vi "Publish Latest Data to Logger.vi"(8 "error in (no error)":errorcluster, 11 "Measurement in":refnum<class "Measurement.lvclass">) -> (0 "error out":errorcluster, 3 "Measurement out":refnum<class "Measurement.lvclass">)   [LabVIEW 2026, in "Measurement Actor.lvlib" / "Measurement.lvclass"]
uses:
  Measurement.lvclass
  Measurement.lvclass/Measurement.ctl
  Logger/Logger Messages/Write Data to File Msg/Write Data to File Msg.lvclass/Write Data to File Msg.ctl
  <vilib>/ActorFramework/Message Enqueuer/Message Enqueuer.lvclass/Message Enqueuer.ctl
  <vilib>/ActorFramework/Message Enqueuer/Enqueue.vi
  Logger/Logger Messages/Write Data to File Msg/Write Data to File Msg.lvclass
  C:/Program Files/National Instruments/LabVIEW 2026/vi.lib/ActorFramework/Message/Message.lvclass
  <vilib>/ActorFramework/Message Priority Queue/Priority Enqueue.vi
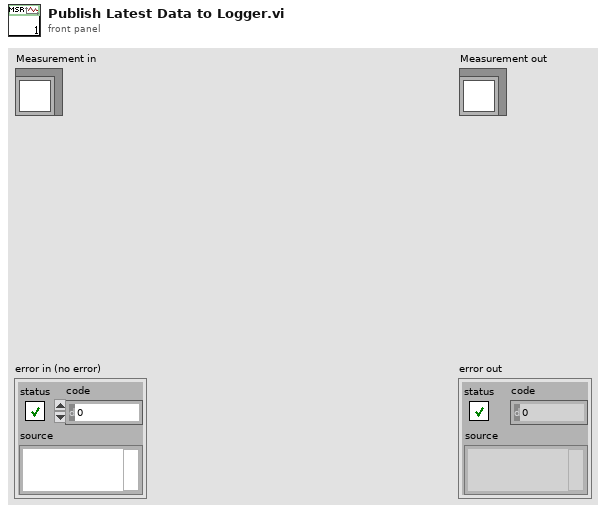
[diagram p1: front panel]
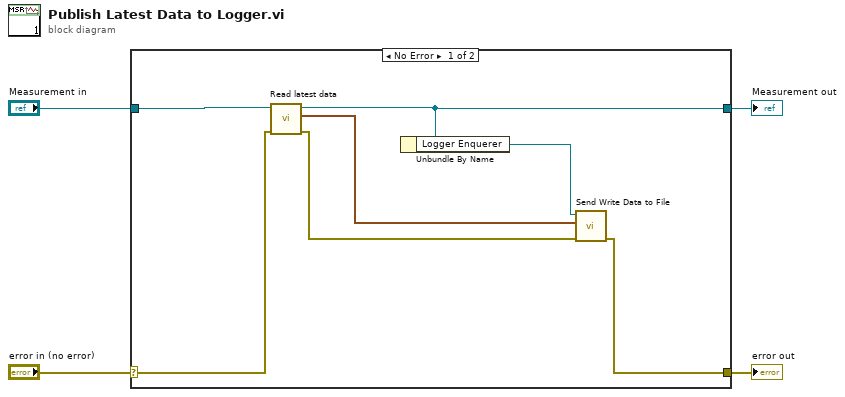
[diagram p0: block diagram]
diagram:
  n1 = case shown="No Error" "error in (no error)" {
    selector: "error in (no error)" -> [w9 w13]
    tunnel: [w5 w13] -> w3
    tunnel: [w10 w12] -> w1
    tunnel: "Measurement in" -> [w11 w12]
    frame No Error {
      n2 = call "Read latest data.vi"("error in (no error)"=w9, "Measurement in"=w11) -> ("error out"=w6:errorcluster, "latest data"=w8:waveform(dbl)[], "Measurement out"=w10:refnum<class "Measurement.lvclass">)  [unwired: 7 in]
      n3 = Unbundle By Name(w10) -> ("Logger Enquerer"=w7:refnum<class "Message Enqueuer.lvclass">)
      n4 = call "Send Write Data to File.vi"("error in (no error)"=w6, "data"=w8, "Message Enqueuer"=w7) -> ("error out"=w5:errorcluster)  [unwired: 7 in, 1 out]
    }
    frame Error {
    }
  }
  "error out" <- w3
  "Measurement out" <- w1
